vi "SolvePnPCore.vi"(5 "Solve PnP Flags":T11, 6 "Camera Parameters":T4, 7 "Use Pose Guess":bool, 8 "error in (no error)":errorcluster, 9 "Pose (Estimate) in":T8, 11 "Point Correspondence Set":T1) -> (0 "error out":errorcluster, 3 "Pose":T8)   [LabVIEW 2020, in "g_ar_toolkit.ar.lvlib"]
uses:
  g_ar_toolkit.ar.lvlib
  SolvePnPFlags.ctl
  Pose.ctl
  rvec.ctl
  g_ar_toolkit.common/tvec.ctl
  Camera Parameters.ctl
  Camera Matrix.ctl
  Camera Distortion Coefficients.ctl
  g_ar_toolkit.common/Image Size (Integer).ctl
  Point Correspondence Set.ctl
  g_ar_toolkit.common/Object Point (Float).ctl
  g_ar_toolkit.common/Image Point (Float).ctl
  bin/g_ar_toolkit.1.32.dll
  g_ar_toolkit.common/g_ar_toolkit.common.lvlib
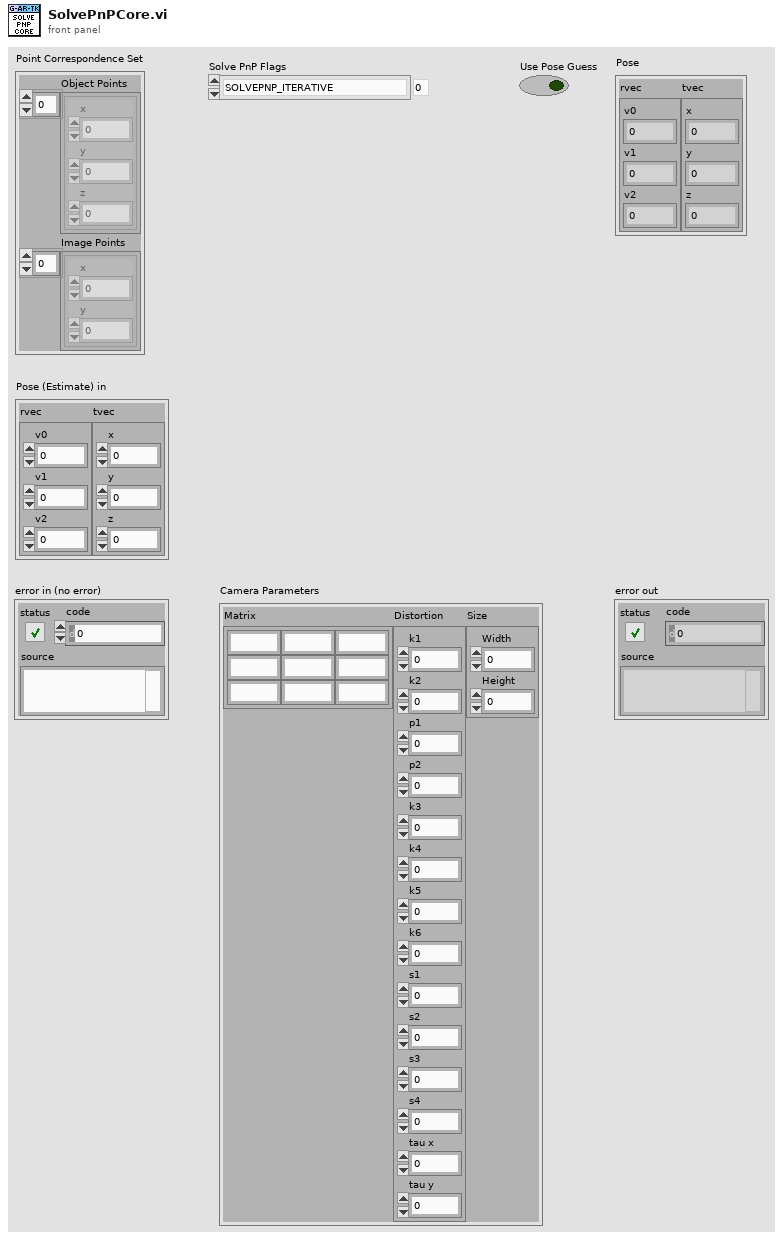
[diagram p1: front panel]
types:
  T1 = typedef "g_ar_toolkit.ar.lvlib/Point Correspondence Set.ctl" = cluster{"Object Points":T2[], "Image Points":T3[]}
  T2 = typedef "g_ar_toolkit.common.lvlib/Object Point (Float).ctl" = cluster{"x":dbl, "y":dbl, "z":dbl}
  T3 = typedef "g_ar_toolkit.common.lvlib/Image Point (Float).ctl" = cluster{"x":dbl, "y":dbl}
  T4 = typedef "g_ar_toolkit.ar.lvlib/Camera Parameters.ctl" = cluster{"Matrix":T5, "Distortion":T6, "Size":T7}
  T5 = typedef "g_ar_toolkit.ar.lvlib/Camera Matrix.ctl" = cluster{"m 0,0":dbl, "m 0,1":dbl, "m 0,2":dbl, "m 1,0":dbl, "m 1,1":dbl, "m 1,2":dbl, "m 2,0":dbl, "m 2,1":dbl, "m 2,2":dbl}
  T6 = typedef "g_ar_toolkit.ar.lvlib/Camera Distortion Coefficients.ctl" = cluster{"k1":dbl, "k2":dbl, "p1":dbl, "p2":dbl, "k3":dbl, "k4":dbl, "k5":dbl, "k6":dbl, "s1":dbl, "s2":dbl, "s3":dbl, "s4":dbl, "tau x":dbl, "tau y":dbl}
  T7 = typedef "g_ar_toolkit.common.lvlib/Image Size (Integer).ctl" = cluster{"Width":u16, "Height":u16}
  T8 = typedef "g_ar_toolkit.ar.lvlib/Pose.ctl" = cluster{"rvec":T9, "tvec":T10}
  T9 = typedef "g_ar_toolkit.ar.lvlib/rvec.ctl" = cluster{"v0":dbl, "v1":dbl, "v2":dbl}
  T10 = typedef "g_ar_toolkit.ar.lvlib/tvec.ctl" = cluster{"x":dbl, "y":dbl, "z":dbl}
  T11 = typedef "g_ar_toolkit.ar.lvlib/SolvePnPFlags.ctl" = enum8{"SOLVEPNP_ITERATIVE", "SOLVEPNP_EPNP", "SOLVEPNP_P3P", "SOLVEPNP_AP3P", "SOLVEPNP_IPPE", "SOLVEPNP_IPPE_SQUARE", "SOLVEPNP_SQPNP"}
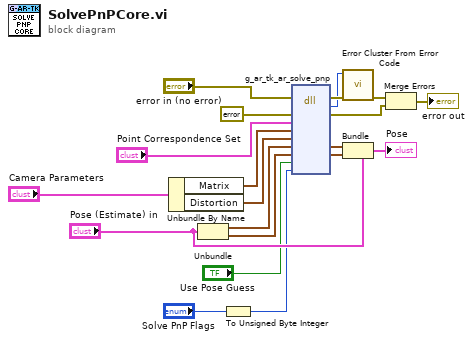
[diagram p0: block diagram]
diagram:
  n1 = Unbundle By Name("Camera Parameters") -> ("Matrix"=w9:T5, "Distortion"=w10:T6)
  n2 = Unbundle("Pose (Estimate) in") -> ("rvec"=w14:T9, "tvec"=w15:T10)
  n3 = To Unsigned Byte Integer(number="Solve PnP Flags") -> (unsigned 8bit integer=w1:u8)
  n4 = dll-call lib="C:/serenial/libraries/g-augmented-reality-toolkit/LabVIEW/bin/g_ar_toolkit.1.*.*" fn="g_ar_tk_ar_solve_pnp" ("g_ar_toolkit.*.*:g_ar_tk_image_copy")(error in="error in (no error)", "error_cluster"=errorcluster {"status"=FALSE, "code"=0, "source"=""} ("error constant"), "corespondence"="Point Correspondence Set", "camera_matrix"=w9, "camera_distortion"=w10, "rvec"=w14, "tvec"=w15, "use_intrinsic"="Use Pose Guess", "flag"=w1) -> (error out=w8:errorcluster, "MgErr"=w7:i32, "error_cluster"=w4:errorcluster, "rvec"=w16:T9, "tvec"=w17:T10)  [unwired: 7 in, 1 out]
  n5 = call <vilib>:"Error Cluster From Error Code.vi"("error in (no error)"=w8, "error code (0)"=w7) -> ("error out"=w6:errorcluster)  [unwired: 7 in]
  n6 = Bundle(cluster="Pose (Estimate) in", "rvec"=w16, "tvec"=w17) -> (→"Pose":T8)
  n7 = Merge Errors(w6, w4) -> (→"error out":errorcluster)
